vi "Simulated Device Page.vi"(8 "error in (no error)":errorcluster, 11 "Node Ptr":T1 format="%.0x") -> (0 "error out":errorcluster)   [LabVIEW 2019, in "J1939 Addon System Explorer.lvlib"]
uses:
  J1939 Addon System Explorer.lvlib
  <vilib>/NI VeriStand/Custom Device API/Custom Device Item Ref.ctl
  Addon Shared/Types/Monitor Settings.ctl
  <vilib>/NI VeriStand/Custom Device API/Custom Device API.lvlib
  Addon Shared/J1939 Addon Shared.lvlib
panel:
  in  "Include DA":bool
  in  "Settings":cluster{"Section Name":string}={"Section Name"="Address Settings"}
  in  "J1939 Name":u64 format="%.0x"
  in  "J1939 Network Address":u8 format="%.0x"
  in  "Description":string
  in  "Name":string
  in  "SHDocVw.IWebBrowser2":refnum<k7>(container)
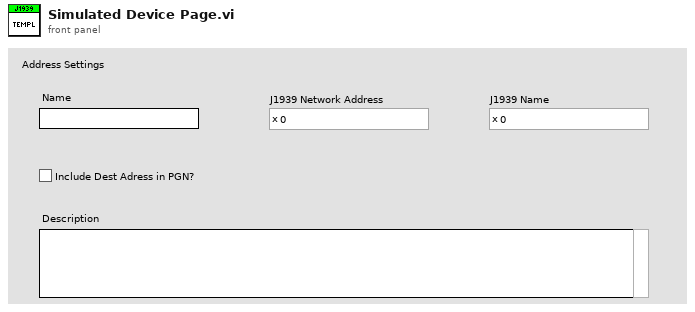
[diagram p1: front panel]
types:
  T1 = typedef "Custom Device API.lvlib/Custom Device Item Ref.ctl" = u64
  T2 = typedef "J1939 Addon Shared.lvlib/Monitor Settings.ctl" = cluster{"Address":u8, "Name":u64, "Include DA":bool}
  T3 = typedef "Custom Device API.lvlib/Custom Device Item Info.ctl" = cluster{"Name":string, "Is Channel":bool, "GUID":string, "Is Waveform":bool}
  T4 = typedef "Custom Device API.lvlib/Custom Device Commands.ctl" = enum16{"Default", "Item renamed", "Shutdown", "Dynamic button pressed"}
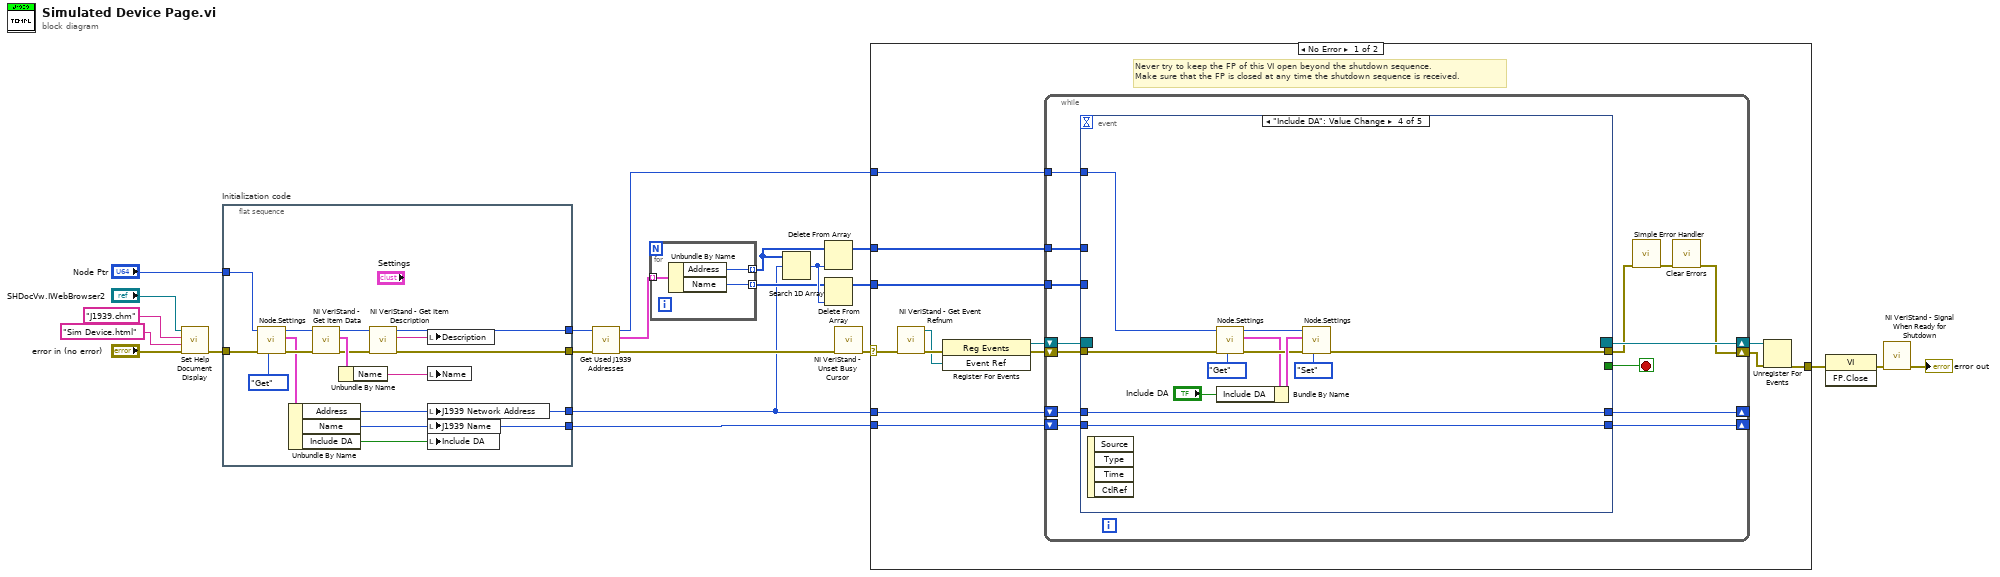
[diagram p0: block diagram]
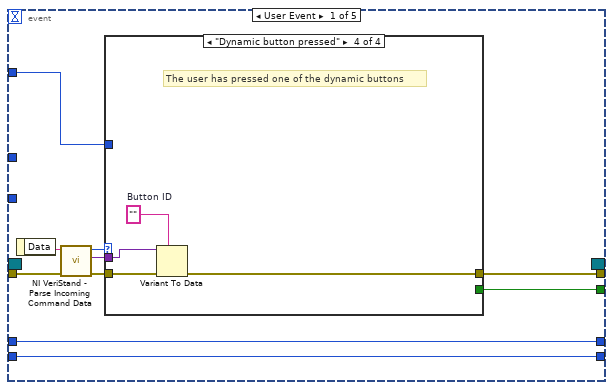
[diagram p2: hidden frame]
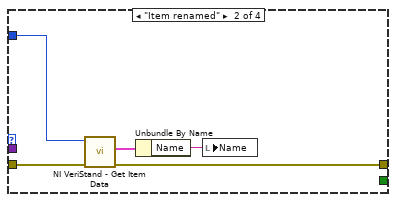
[diagram p4: hidden frame]
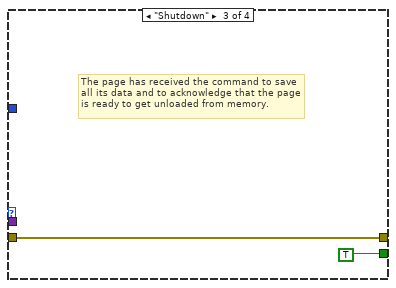
[diagram p5: hidden frame]
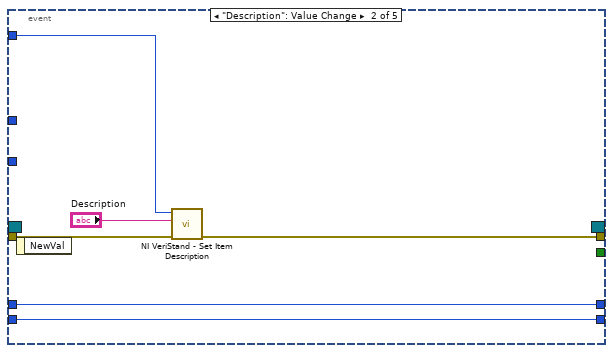
[diagram p6: hidden frame]
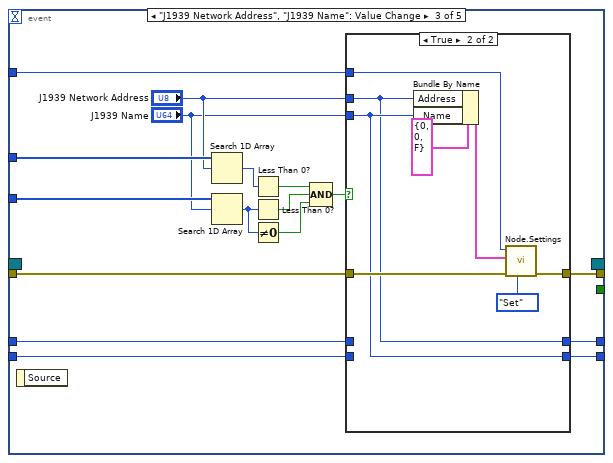
[diagram p7: hidden frame]
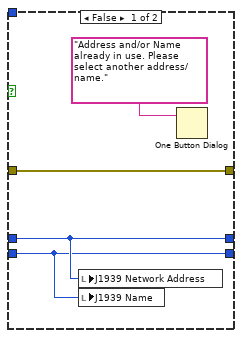
[diagram p8: hidden frame]
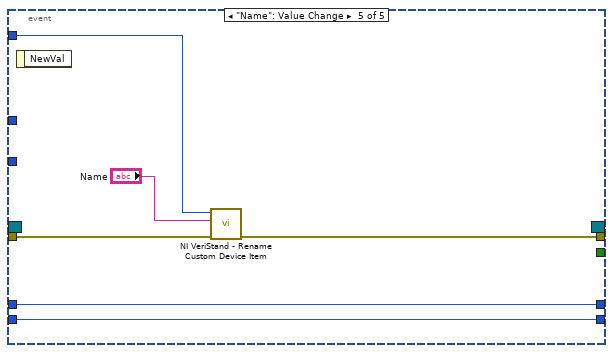
[diagram p9: hidden frame]
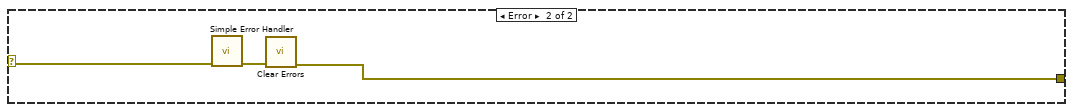
[diagram p10: hidden frame]
diagram:
  n1 = call "Set Help Document Display.vi"("error in (no error)"="error in (no error)", "HTML File"="Sim Device.html", "Main CHM File"="J1939.chm", "SHDocVw.IWebBrowser2"="SHDocVw.IWebBrowser2") -> ("error out"=w13:errorcluster)  [unwired: 7 in]
  n2 = flat-sequence "Initialization code" {
    tunnel: w13 -> [w31]
    tunnel: "Node Ptr" -> [w30]
    tunnel: [w35] -> w11
    tunnel: [w33] -> w9
    tunnel: [w26] -> w3
    tunnel: [w25] -> w8
    frame #0 {
      n3 = call "Node.Settings.vi"("Action"=enum8{"Get", "Set"}."Get", "error in (no error)"=w31, "Item Ref in"=w30) -> ("error out"=w28:errorcluster, "Node.Settings"=w27:T2, "Item Ref out"=w29:T1)  [unwired: 6 in]
      n4 = Unbundle By Name(w27) -> ("Address"=w26:u8, "Name"=w25:u64, "Include DA"=w23:bool)
      n5 = call <vilib>:"NI VeriStand - Get Item Data.vi"("error in (no error)"=w28, "Item Ref in"=w29) -> ("error out"=w36:errorcluster, "Item Info"=w38:T3, "Item Ref out"=w34:T1)  [unwired: 7 out]
      n6 = Unbundle By Name(w38) -> ("Name"=w37:string)
      n7 = call <vilib>:"NI VeriStand - Get Item Description.vi"("error in (no error)"=w36, "Item Ref in"=w34) -> ("error out"=w35:errorcluster, "Description"=w32:string, "Item Ref out"=w33:T1)  [unwired: 6 in, 1 out]
      n8 = local write "Description"(w32) -> ()
      n9 = local write "Name"(w37) -> ()
      n10 = local write "J1939 Network Address"(w26) -> ()
      n11 = local write "J1939 Name"(w25) -> ()
      n12 = local write "Include DA"(w23) -> ()
    }
  }
  n13 = call "Get Used J1939 Addresses.vi"("error in (no error)"=w11, "Node Ptr"=w9) -> ("error out"=w12:errorcluster, "Nodes"=w4:T2[], "Item Ref out"=w10:T1)  [unwired: 7 in]
  n14 = for {
    tunnel: w4 -> [w41] mode=indexing
    tunnel: [w40] -> w7 mode=indexing
    tunnel: [w39] -> w5 mode=indexing
    n15 = Unbundle By Name(w41) -> ("Address"=w40:u8, "Name"=w39:u64)
  }
  n16 = Search 1D Array(1D array=w7, element=w3) -> (index of element=w6:i32)  [unwired: 1 in]
  n17 = Delete From Array(array=w7, index=w6) -> (array with subset deleted=w2:u8[])  [unwired: 1 in, 1 out]
  n18 = Delete From Array(array=w5, index=w6) -> (array with subset deleted=w1:u64[])  [unwired: 1 in, 1 out]
  n19 = call <vilib>:"NI VeriStand - Unset Busy Cursor.vi"("error in (no error)"=w12) -> ("error out"=w18:errorcluster)  [unwired: 10 out]
  n20 = case shown="No Error" w18 {
    selector: w18 -> [w46 w146]
    tunnel: [w51 w144] -> w22
    tunnel: w10 -> [w47 _]
    tunnel: w3 -> [w45 _]
    tunnel: w8 -> [w44 _]
    tunnel: w2 -> [w43 _]
    tunnel: w1 -> [w42 _]
    frame No Error {
      # "Never try to keep the FP of this VI open beyond the shutdown sequence.\nMake sure that the FP is closed at any time the shutdown sequence is received."
      n21 = call <vilib>:"NI VeriStand - Get Event Refnum.vi"("error in (no error)"=w46) -> ("error out"=w54:errorcluster, "Event Ref"=w50:refnum<user-event>)  [unwired: 9 out]
      n22 = register-events(error in=w54, w50) -> (reference out=w48:refnum<event-registration>, error out=w49:errorcluster)  [unwired: 1 in]
      n23 = while {
        tunnel: w47 -> [w64]
        shift-right: [w61] -> w52
        shift-left: w49 -> [w67]
        shift-right: [w68] -> w53
        shift-left: w48 -> [w66]
        tunnel: w43 -> [w58]
        tunnel: w42 -> [w57]
        shift-right: [w56] -> _
        shift-left: w45 -> [w60]
        shift-right: [w55] -> _
        shift-left: w44 -> [w59]
        stop <- w65 stop-if-true
        n24 = event shown="[3] \"Include DA\": Value Change" {
          selector: w66 -> [_ _ _ _ _]
          dyn-events: [_ _ _ _ _] -> w68
          timeout: _ -> [_ _ _ _ _]
          tunnel: w67 -> [w78 w96 w113 w130 w143]
          tunnel: [w74 _ _ _ _] -> w65
          tunnel: [w73 w93 w112 w137 w141] -> w63
          tunnel: w64 -> [w72 w94 w111 w129 w142]
          tunnel: w60 -> [w69 w91 w110 w133 w138]
          tunnel: w59 -> [w70 w92 w109 w134 w139]
          tunnel: w58 -> [_ _ w103 _ _]
          tunnel: w57 -> [_ _ w102 _ _]
          tunnel: [w69 w91 w98 w133 w138] -> w56
          tunnel: [w70 w92 w97 w134 w139] -> w55
          event User Event {
            n25 = event-data() -> ("Data"=w77:string)  [unwired: 1 out]
            n26 = call <vilib>:"NI VeriStand - Parse Incoming Command Data.vi"("error in (no error)"=w78, "Incoming data"=w77) -> ("error out"=w76:errorcluster, "Outgoing data"=w71:variant, "Action"=w75:T4)  [unwired: 7 out]
            n27 = case shown="\"Dynamic button pressed\"" w75 {
              tunnel: w76 -> [w79 w82 w85 w90]
              tunnel: [_ _ TRUE _] -> w74
              tunnel: [w79 w80 w85 w87] -> w73
              tunnel: w72 -> [_ w81 _ _]
              tunnel: w71 -> [_ _ _ w89]
              frame "Default", Default {
              }
              frame "Item renamed" {
                n28 = call <vilib>:"NI VeriStand - Get Item Data.vi"("error in (no error)"=w82, "Item Ref in"=w81) -> ("error out"=w80:errorcluster, "Item Info"=w83:T3)  [unwired: 8 out]
                n29 = Unbundle By Name(w83) -> ("Name"=w84:string)
                n30 = local write "Name"(w84) -> ()
              }
              frame "Shutdown" {
                # "The page has received the command to save all its data and to acknowledge that the page is ready to get unloaded from memory."
              }
              frame "Dynamic button pressed" {
                w88 = ""  # Button ID
                # "The user has pressed one of the dynamic buttons"
                n31 = Variant To Data(error in=w90, type=w88, Variant=w89) -> (error out=w87:errorcluster)  [unwired: 1 out]
              }
            }
          }
          event "Description": Value Change {
            n32 = event-data() -> ()  [unwired: 2 out]
            n33 = call <vilib>:"NI VeriStand - Set Item Description.vi"("error in (no error)"=w96, "Description"="Description", "Item Ref in"=w94) -> ("error out"=w93:errorcluster)  [unwired: 6 in, 2 out]
          }
          event "J1939 Network Address", "J1939 Name": Value Change {
            n34 = event-data() -> ()  [unwired: 2 out]
            n35 = Search 1D Array(1D array=w103, element="J1939 Network Address") -> (index of element=w106:i32)  [unwired: 1 in]
            n36 = Search 1D Array(1D array=w102, element="J1939 Name") -> (index of element=w105:i32)  [unwired: 1 in]
            n37 = Less Than 0?(x=w106) -> (x < 0?=w108:bool)
            n38 = Less Than 0?(x=w105) -> (x < 0?=w107:bool)
            n39 = Not Equal To 0?(x=w105) -> (x != 0?=w104:bool)
            n40 = Compound Arithmetic op=AND(w108, w107, w104) -> (w99:bool)
            n41 = case shown="True" w99 {
              tunnel: "J1939 Name" -> [_ w121]
              tunnel: w113 -> [w117 w124]
              tunnel: [w117 w123] -> w112
              tunnel: w111 -> [_ w122]
              tunnel: "J1939 Network Address" -> [_ w120]
              tunnel: w110 -> [w115 _]
              tunnel: w109 -> [w114 _]
              tunnel: [w115 w120] -> w98
              tunnel: [w114 w121] -> w97
              frame False {
                n42 = local write "J1939 Network Address"(w115) -> ()
                n43 = local write "J1939 Name"(w114) -> ()
                n44 = One Button Dialog(message="Address and/or Name already in use. Please select another address/name.") -> ()  [unwired: 1 in, 1 out]
              }
              frame True {
                n45 = Bundle By Name(cluster=T2 {"Address"=0, "Name"=0, "Include DA"=FALSE} ("J1939 XNET Settings"), "Address"=w120, "Name"=w121) -> (w119:T2)
                n46 = call "Node.Settings.vi"("Action"=enum8{"Get", "Set"}."Set", "error in (no error)"=w124, "Node.Settings"=w119, "Item Ref in"=w122) -> ("error out"=w123:errorcluster)  [unwired: 5 in, 2 out]
              }
            }
          }
          event "Include DA": Value Change {
            n47 = event-data() -> ()  [unwired: 5 out]
            n48 = call "Node.Settings.vi"("Action"=enum8{"Get", "Set"}."Get", "error in (no error)"=w130, "Item Ref in"=w129) -> ("error out"=w131:errorcluster, "Node.Settings"=w127:T2, "Item Ref out"=w128:T1)  [unwired: 6 in]
            n49 = Bundle By Name(cluster=w127, "Include DA"="Include DA") -> (w136:T2)
            n50 = call "Node.Settings.vi"("Action"=enum8{"Get", "Set"}."Set", "error in (no error)"=w131, "Node.Settings"=w136, "Item Ref in"=w128) -> ("error out"=w137:errorcluster)  [unwired: 5 in, 2 out]
          }
          event "Name": Value Change {
            n51 = event-data() -> ()  [unwired: 2 out]
            n52 = call <vilib>:"NI VeriStand - Rename Custom Device Item.vi"("error in (no error)"=w143, "New Name"="Name", "Item Ref in"=w142) -> ("error out"=w141:errorcluster)  [unwired: 1 in, 7 out]
          }
        }
        n53 = call <vilib>:"Simple Error Handler.vi"("error in (no error)"=w63) -> ("error out"=w62:errorcluster)  [unwired: 1 in, 7 out]
        n54 = call <vilib>:"Clear Errors.vi"("error in (no error)"=w62) -> ("error out"=w61:errorcluster)  [unwired: 1 in, 5 out]
      }
      n55 = Unregister For Events(event registration refnum=w53, error in=w52) -> (error out=w51:errorcluster)
    }
    frame Error {
      n56 = call <vilib>:"Simple Error Handler.vi"("error in (no error)"=w146) -> ("error out"=w145:errorcluster)  [unwired: 1 in, 7 out]
      n57 = call <vilib>:"Clear Errors.vi"("error in (no error)"=w145) -> ("error out"=w144:errorcluster)  [unwired: 1 in, 5 out]
    }
  }
  n58 = invoke class="VI" method="FP.Close"(error in=w22) -> (error out=w21:errorcluster)  [unwired: 2 in, 2 out]
  n59 = call <vilib>:"NI VeriStand - Signal When Ready for Shutdown.vi"("error in (no error)"=w21) -> ("error out"=→"error out":errorcluster)  [unwired: 10 out]
